vi "Vector fun.vi"() -> ()   [LabVIEW 2024]
panel:
  in  "vectors":T1(array[cluster]) {"Y origin" scale=0.0..100.0; "X origin" scale=0.0..100.0; "vector"."length" format="%.1f"; "vector"."angle" format="%.1f"}
  out "2D Picture":picture
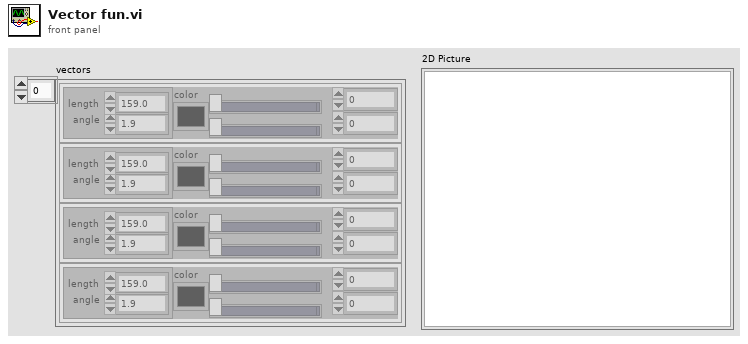
[diagram p1: front panel]
types:
  T1 = cluster{"vector":cluster{"length":dbl, "angle":dbl}, "color":u32, "X origin":i16, "Y origin":i16}[]
  T2 = cluster{"Width":u16, "Style":enum32{"Solid", "Dash", "Dot", "DashDot", "DashDotDot"}}
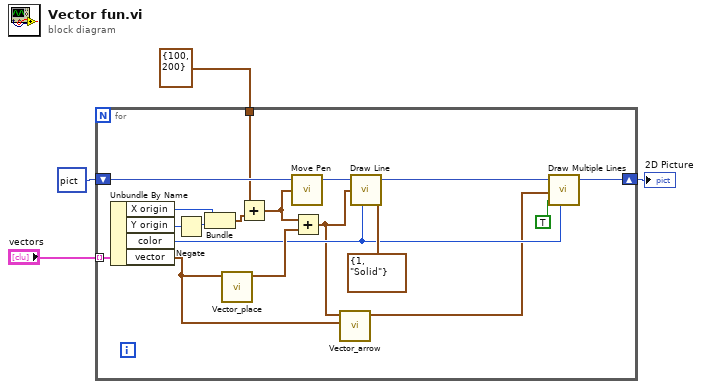
[diagram p0: block diagram]
diagram:
  n1 = for {
    tunnel: "vectors" -> [w19] mode=indexing
    shift-right: [w10] -> w4
    shift-left: picture data[5B] ("new picture") -> [w18]
    tunnel: cluster{"x":i16, "y":i16} {"x"=100, "y"=200} ("new position") -> [w13]
    n2 = Unbundle By Name(w19) -> ("X origin"=w15:i16, "Y origin"=w17:i16, "color"=w9:u32, "vector"=w8:cluster{"length":dbl, "angle":dbl})
    n3 = Negate(x=w17) -> (-x=w16:i16)
    n4 = Bundle("X origin"=w15, w16) -> (w14:cluster{"X origin":i16, i16})  [unwired: 1 in]
    n5 = call "Vector_place.vi"("vector"=w8) -> ("x,y"=w20:cluster{dbl, dbl})  [unwired: 10 in]
    n6 = Add(x=w13, y=w14) -> (x+y=w12:cluster{i16, i16})
    n7 = call <vilib>:"Move Pen.vi"("new position"=w12, "picture"=w18) -> ("new picture"=w22:picture)  [unwired: 3 in]
    n8 = Add(x=w12, y=w20) -> (x+y=w6:cluster{dbl, dbl})
    n9 = call "Vector_arrow.vi"("vector"=w8, "tip"=w6) -> ("(x,y)"=w7:cluster{dbl, dbl}[])  [unwired: 9 in]
    n10 = call <vilib>:"Draw Line.vi"("picture"=w22, "end point"=w6, "color(black)"=w9, "pen"=T2 {"Width"=1, "Style"=enum."Solid"}) -> ("new picture"=w11:picture)  [unwired: 5 in]
    n11 = call <vilib>:"Draw Multiple Lines.vi"("picture"=w11, "line endpoints"=w7, "fill?(F)"=TRUE, "color(black)"=w9) -> ("new picture"=w10:picture)  [unwired: 5 in]
  }
  "2D Picture" <- w4
